vi "G-Sensitivity.vi"() -> ()   [LabVIEW 2023]
uses:
  <vilib>/addons/database/Connection.llb/DB Tools Open Connec (String).vi
  <vilib>/regexp/Match Regular Expression.xnode
  <vilib>/addons/database/NI_Database_API.lvlib
panel:
  out "Total Gamma (ppb/g)":dbl
  out "Y (ppb/g)":dbl
  out "Z (ppb/g)":dbl
  out "X (ppb/g)":dbl
  in  "Peak G Vib Level":dbl
  in  "Freq Vibe":dbl
  in  "Freq (MHz)":dbl
  in  "Y Value (dBc)":dbl
  in  "Z Value (dBc)":dbl
  in  "X Value (dBc)":dbl
  in  "DC_SN":string
  out "TimeRun":string
  in  "Exit":bool
  in  "Enter":bool
  in  "Work Order":string
  in  "Employee Number":string
  # "G-Sensitivity Data Logger"
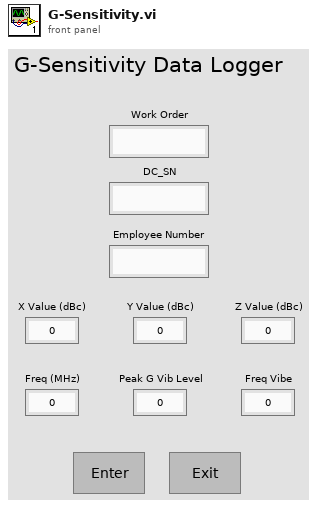
[diagram p1: front panel]
types:
  T1 = typedef "NI_Database_API.lvlib/Conn ObjectReference.ctl" = refnum<k1>
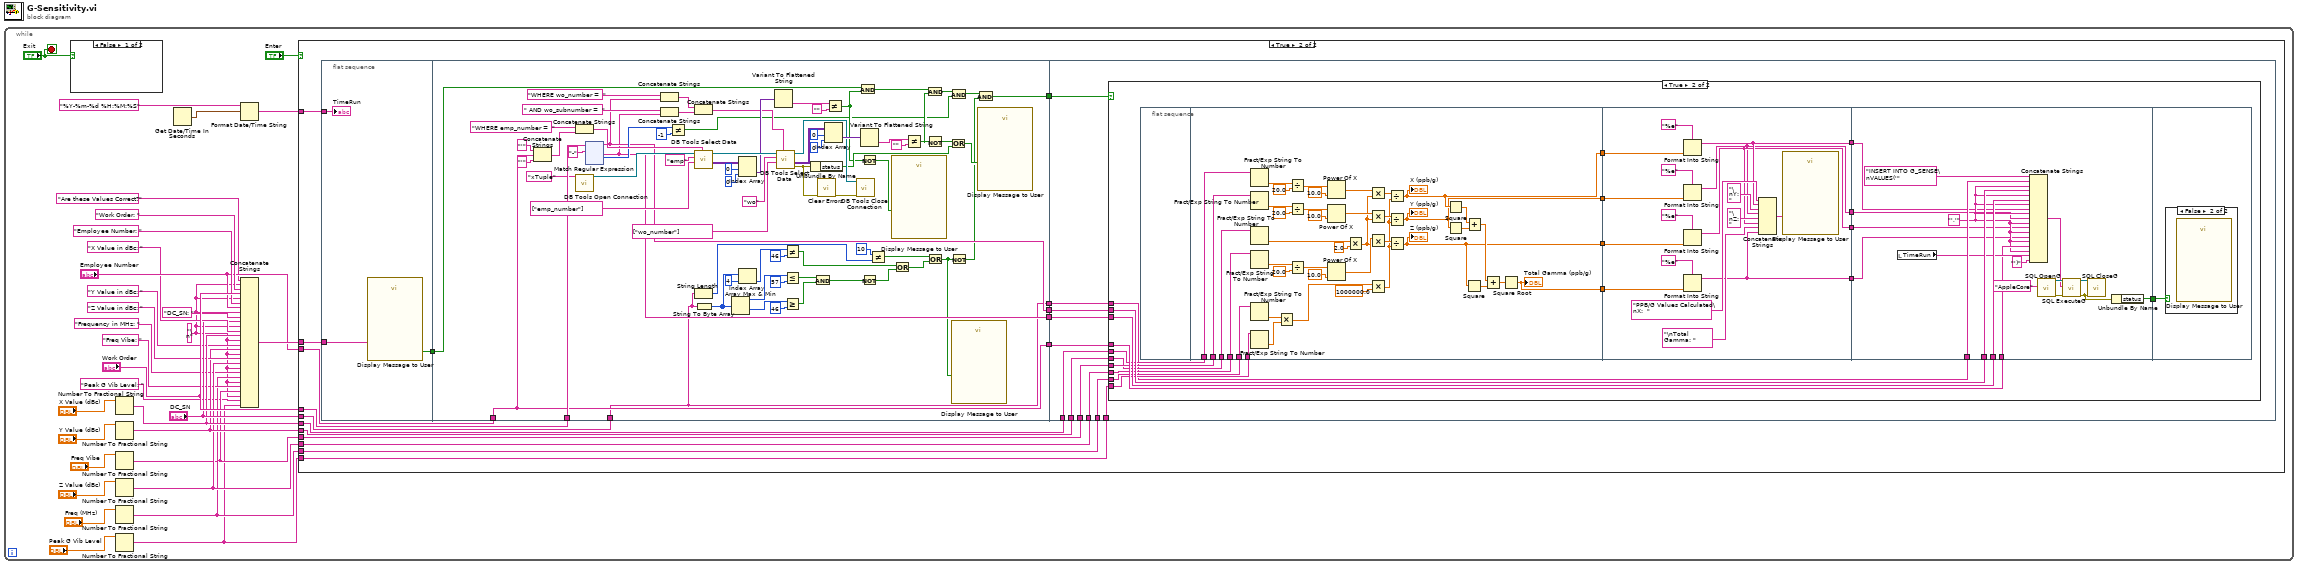
[diagram p0: block diagram]
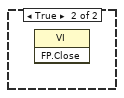
[diagram p2: hidden frame]
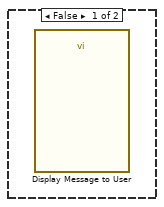
[diagram p4: hidden frame]
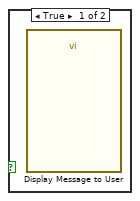
[diagram p5: hidden frame]
diagram:
  n1 = while {
    stop <- "Exit" stop-if-true
    w1 = "\n" ("string")
    n2 = case shown="False" "Exit" {
      frame False {
      }
      frame True {
        n3 = invoke class="VI" method="FP.Close"() -> ()  [unwired: 3 in, 3 out]
      }
    }
    n4 = Number To Fractional String(number="X Value (dBc)") -> (F-format string=w20:string)  [unwired: 3 in]
    n5 = Number To Fractional String(number="Y Value (dBc)") -> (F-format string=w14:string)  [unwired: 3 in]
    n6 = Number To Fractional String(number="Freq Vibe") -> (F-format string=w6:string)  [unwired: 3 in]
    n7 = Number To Fractional String(number="Z Value (dBc)") -> (F-format string=w13:string)  [unwired: 3 in]
    n8 = Number To Fractional String(number="Freq (MHz)") -> (F-format string=w7:string)  [unwired: 3 in]
    n9 = Number To Fractional String(number="Peak G Vib Level") -> (F-format string=w5:string)  [unwired: 3 in]
    n10 = Get Date/Time In Seconds() -> (seconds since 1Jan1904=w23:timestamp)
    n11 = Format Date/Time String(time format string (%c)="%Y-%m-%d %H:%M:%S", seconds (now)=w23) -> (date/time string=w22:string)  [unwired: 1 in]
    n12 = Concatenate Strings("Are these Values Correct?" ("string"), w1, "Work Order: " ("string"), "Work Order", w1, "Employee Number: " ("string"), "Employee Number", w1, "DC_SN: " ("string"), "DC_SN", w1, "X Value in dBc: " ("string"), w20, w1, "Y Value in dBc: " ("string"), w14, w1, "Z Value in dBc: " ("string"), w13, w1, "Frequency in MHz: " ("string"), w7, w1, "Freq Vibe: " ("string"), w6, w1, "Peak G Vib Level: " ("string"), w5) -> (w31:string)
    n13 = case shown="True" "Enter" {
      tunnel: w31 -> [_ w49]
      tunnel: "Work Order" -> [_ w47]
      tunnel: "Employee Number" -> [_ w46]
      tunnel: w22 -> [_ w44]
      tunnel: "DC_SN" -> [_ w40]
      tunnel: w20 -> [_ w39]
      tunnel: w14 -> [_ w38]
      tunnel: w13 -> [_ w37]
      tunnel: w5 -> [_ w36]
      tunnel: w7 -> [_ w35]
      tunnel: w6 -> [_ w34]
      frame False {
      }
      frame True {
        n14 = flat-sequence {
          tunnel: [w52] -> w48
          tunnel: w49 -> [w51]
          tunnel: w44 -> [w50]
          tunnel: w48 -> [w80]
          tunnel: [w54] -> w45
          tunnel: w47 -> [w111]
          tunnel: w46 -> [w77]
          tunnel: [w79] -> w43
          tunnel: [w78] -> w42
          tunnel: [w77] -> w41
          tunnel: w40 -> [w74]
          tunnel: [w74] -> w33
          tunnel: w45 -> [w251]
          tunnel: w43 -> [w250]
          tunnel: w42 -> [w249]
          tunnel: w41 -> [w248]
          tunnel: w39 -> [w247]
          tunnel: w38 -> [w246]
          tunnel: w37 -> [w245]
          tunnel: w36 -> [w244]
          tunnel: w35 -> [w243]
          tunnel: w34 -> [w242]
          tunnel: w33 -> [w241]
          frame #0 {
            n15 = call "Display Message to User"("Message"=w51) -> ("Yes"=w52:bool)  [unwired: 9 in, 1 out]
            "TimeRun" <- w50
          }
          frame #1 {
            n16 = Concatenate Strings("'" ("string"), w77, "'" ("string")) -> (w93:string)
            n17 = Concatenate Strings("WHERE emp_number =  " ("condition"), w93) -> (w115:string)
            n18 = call-poly <vilib>:"DB Tools Open Connection.vi"("connection information"="xTuple" ("Connection Strings")) -> ("connection reference"=w114:T1)  [unwired: 7 in, 1 out]
            n19 = xnode "Match Regular Expression"("input string"=w111, "regular expression"="-") -> ("before match"=w79:string, "after match"=w78:string, "offset past match"=w92:i32)  [unwired: 4 in, 2 out]
            n20 = Concatenate Strings("WHERE wo_number =  " ("condition"), w79) -> (w88:string)
            n21 = Concatenate Strings(" AND wo_subnumber =  " ("condition"), w78) -> (w89:string)
            n22 = Not Equal?(x=w92, y=-1) -> (x != y?=w75:bool)
            n23 = Concatenate Strings(w88, w89) -> (w90:string)
            n24 = call <vilib>:"DB Tools Select Data.vi"("condition"=w115, "columns"=string[] ["emp_number"], "table"="emp", "connection reference"=w114) -> ("data"=w117:variant[][], "connection reference out"=w120:T1)  [unwired: 2 in, 1 out]
            n25 = String Length(string=w74) -> (length=w64:i32)
            n26 = String To Byte Array(string=w74) -> (unsigned byte array=w67:u8[])
            n27 = Array Max & Min(array=w67) -> (max value=w69:u8, min value=w68:u8)  [unwired: 2 out]
            n28 = Index Array(array=w117, index (row)=0, index (col)=0 ("disabled index (col)")) -> (element=w116:variant)
            n29 = Index Array(array=w67, index=4) -> (element=w65:u8)
            n30 = Variant To Flattened String(Variant=w116) -> (data string=w118:string)  [unwired: 1 out]
            n31 = call <vilib>:"DB Tools Select Data.vi"("condition"=w90, "columns"=string[] ["wo_number"], "table"="wo", "connection reference"=w120) -> ("error out"=w86:errorcluster, "data"=w123:variant[][], "connection reference out"=w87:T1)  [unwired: 2 in]
            n32 = Not Equal?(x=w65, y=u8 46) -> (x != y?=w66:bool)
            n33 = Less Or Equal?(x=w69, y=u8 57) -> (x <= y?=w70:bool)
            n34 = Greater Or Equal?(x=w68, y=u8 46) -> (x >= y?=w71:bool)
            n35 = Unbundle By Name(w86) -> ("status"=w83:bool)
            n36 = And(x=w70, y=w71) -> (x .and. y?=w72:bool)
            n37 = call <vilib>:"Clear Errors.vi"("error in (no error)"=w86) -> ("error out"=w85:errorcluster)  [unwired: 5 in, 1 out]
            n38 = Index Array(array=w123, index (row)=0, index (col)=0 ("disabled index (col)")) -> (element=w121:variant)
            n39 = Not Equal?(x=w118, y="") -> (x != y?=w81:bool)
            n40 = call <vilib>:"DB Tools Close Connection.vi"("error in (no error)"=w85, "connection reference"=w87) -> ()  [unwired: 5 in, 1 out]
            n41 = And(x=w80, y=w81) -> (x .and. y?=w98:bool)
            n42 = Variant To Flattened String(Variant=w121) -> (data string=w122:string)  [unwired: 1 out]
            n43 = Not(x=w81) -> (.not. x?=w119:bool)
            n44 = Not(x=w72) -> (.not. x?=w73:bool)
            n45 = Not Equal?(x=10, y=w64) -> (x != y?=w57:bool)
            n46 = call "Display Message to User"("Enable"=w119) -> ()  [unwired: 9 in, 2 out]
            n47 = Or(x=w66, y=w73) -> (x .or. y?=w58:bool)
            n48 = Not Equal?(x=w122, y="") -> (x != y?=w97:bool)
            n49 = And(x=w98, y=w97) -> (x .and. y?=w76:bool)
            n50 = Not(x=w97) -> (.not. x?=w84:bool)
            n51 = Or(x=w57, y=w58) -> (x .or. y?=w56:bool)
            n52 = Or(x=w84, y=w83) -> (x .or. y?=w82:bool)
            n53 = And(x=w76, y=w75) -> (x .and. y?=w55:bool)
            n54 = Not(x=w56) -> (.not. x?=w53:bool)
            n55 = call "Display Message to User"("Enable"=w56) -> ()  [unwired: 9 in, 2 out]
            n56 = And(x=w55, y=w53) -> (x .and. y?=w54:bool)
            n57 = call "Display Message to User"("Enable"=w82) -> ()  [unwired: 9 in, 2 out]
          }
          frame #2 {
            n58 = case shown="True" w251 {
              tunnel: w250 -> [_ w270]
              tunnel: w249 -> [_ w269]
              tunnel: w248 -> [_ w268]
              tunnel: w247 -> [_ w267]
              tunnel: w246 -> [_ w266]
              tunnel: w245 -> [_ w265]
              tunnel: w244 -> [_ w264]
              tunnel: w243 -> [_ w263]
              tunnel: w242 -> [_ w262]
              tunnel: w241 -> [_ w252]
              frame False {
                n59 = call "Display Message to User"() -> ()  [unwired: 10 in, 2 out]
              }
              frame True {
                n60 = flat-sequence {
                  tunnel: w267 -> [w311]
                  tunnel: w266 -> [w310]
                  tunnel: w265 -> [w309]
                  tunnel: w264 -> [w308]
                  tunnel: w263 -> [w307]
                  tunnel: w262 -> [w306]
                  tunnel: [w274] -> w261
                  tunnel: [w273] -> w260
                  tunnel: [w272] -> w259
                  tunnel: [w271] -> w258
                  tunnel: w261 -> [w322]
                  tunnel: w260 -> [w313]
                  tunnel: w259 -> [w319]
                  tunnel: w258 -> [w316]
                  tunnel: [w318] -> w256
                  tunnel: [w315] -> w255
                  tunnel: [w312] -> w254
                  tunnel: [w323] -> w253
                  tunnel: w252 -> [w346]
                  tunnel: w270 -> [w345]
                  tunnel: w269 -> [w344]
                  tunnel: w268 -> [w341]
                  tunnel: [w339] -> w257
                  tunnel: w256 -> [w338]
                  tunnel: w255 -> [w337]
                  tunnel: w254 -> [w336]
                  tunnel: w253 -> [w335]
                  tunnel: w257 -> [w348]
                  frame #0 {
                  }
                  frame #1 {
                    n61 = Fract/Exp String To Number(string=w311) -> (number=w303:dbl)  [unwired: 3 in, 1 out]
                    n62 = Fract/Exp String To Number(string=w310) -> (number=w290:dbl)  [unwired: 3 in, 1 out]
                    n63 = Fract/Exp String To Number(string=w306) -> (number=w304:dbl)  [unwired: 3 in, 1 out]
                    n64 = Fract/Exp String To Number(string=w309) -> (number=w291:dbl)  [unwired: 3 in, 1 out]
                    n65 = Fract/Exp String To Number(string=w307) -> (number=w298:dbl)  [unwired: 3 in, 1 out]
                    n66 = Fract/Exp String To Number(string=w308) -> (number=w297:dbl)  [unwired: 3 in, 1 out]
                    n67 = Multiply(x=w298, y=w297) -> (x*y=w296:dbl)
                    n68 = Divide(x=w303, y=20.0) -> (x/y=w300:dbl)
                    n69 = Divide(x=w290, y=20.0) -> (x/y=w288:dbl)
                    n70 = Divide(x=w291, y=20.0) -> (x/y=w286:dbl)
                    n71 = Power Of X(1:10.0 ("x"), 2:w300) -> (0:w299:dbl)
                    n72 = Power Of X(1:10.0 ("x"), 2:w288) -> (0:w285:dbl)
                    n73 = Power Of X(1:10.0 ("x"), 2:w286) -> (0:w284:dbl)
                    n74 = Multiply(x=w304, y=2.0) -> (x*y=w283:dbl)
                    n75 = Multiply(x=w299, y=w283) -> (x*y=w294:dbl)
                    n76 = Multiply(x=w285, y=w283) -> (x*y=w281:dbl)
                    n77 = Multiply(x=w284, y=w283) -> (x*y=w282:dbl)
                    n78 = Multiply(x=w296, y=1000000.0) -> (x*y=w280:dbl)
                    n79 = Divide(x=w294, y=w280) -> (x/y=w274:dbl)
                    "X (ppb/g)" <- w274
                    n80 = Divide(x=w281, y=w280) -> (x/y=w273:dbl)
                    "Y (ppb/g)" <- w273
                    n81 = Divide(x=w282, y=w280) -> (x/y=w272:dbl)
                    "Z (ppb/g)" <- w272
                    n82 = Square(x=w274) -> (x^2=w279:dbl)
                    n83 = Square(x=w273) -> (x^2=w278:dbl)
                    n84 = Square(x=w272) -> (x^2=w276:dbl)
                    n85 = Add(x=w279, y=w278) -> (x+y=w277:dbl)
                    n86 = Add(x=w277, y=w276) -> (x+y=w275:dbl)
                    n87 = Square Root(x=w275) -> (sqrt(x)=w271:dbl)
                    "Total Gamma (ppb/g)" <- w271
                  }
                  frame #2 {
                    n88 = Format Into String(format string="%e", w322) -> (resulting string=w323:string)  [unwired: 2 in, 1 out]
                    n89 = Format Into String(format string="%e", w313) -> (resulting string=w312:string)  [unwired: 2 in, 1 out]
                    n90 = Format Into String(format string="%e", w319) -> (resulting string=w318:string)  [unwired: 2 in, 1 out]
                    n91 = Format Into String(format string="%e", w316) -> (resulting string=w315:string)  [unwired: 2 in, 1 out]
                    n92 = Concatenate Strings("PPB/G Values Calculated\nX:  " ("string"), w323, "\nY: " ("string"), w312, "\nZ: " ("string"), w318, "\nTotal Gamma: " ("string"), w315) -> (w325:string)
                    n93 = call "Display Message to User"("Message"=w325) -> ()  [unwired: 9 in, 2 out]
                  }
                  frame #3 {
                    w340 = "','" ("string")
                    n94 = local read "TimeRun"() -> (w342:string)
                    n95 = Concatenate Strings("INSERT INTO G_SENSE\nVALUES('" ("string"), w346, w340, w345, w340, w344, w340, w335, w340, w336, w340, w338, w340, w337, w340, w341, w340, w342, "')" ("string")) -> (w331:string)
                    n96 = call "SQL OpenG.vi"("ConnectionString In"="AppleCore") -> ("Connection Out"=w333:refnum<k7>, "Error out"=w332:errorcluster)  [unwired: 17 in]
                    n97 = call "SQL ExecuteG.vi"("Connection In"=w333, "SQL Query"=w331, "Error in (no error)"=w332) -> ("Connection Out"=w330:refnum<k7>, "Error out"=w329:errorcluster)  [unwired: 15 in]
                    n98 = call "SQL CloseG.vi"("Connection In"=w330, "Error in (no error)"=w329) -> ()  [unwired: 17 in, 1 out]
                    n99 = Unbundle By Name(w329) -> ("status"=w339:bool)
                  }
                  frame #4 {
                    n100 = case shown="False" w348 {
                      frame True {
                        n101 = call "Display Message to User"() -> ()  [unwired: 10 in, 2 out]
                      }
                      frame False {
                        n102 = call "Display Message to User"() -> ()  [unwired: 10 in, 2 out]
                      }
                    }
                  }
                }
              }
            }
          }
        }
      }
    }
  }
